vi "Boolean State Change.vi"(11 "Bool In":bool) -> (3 "State Change?":bool)   [LabVIEW 2018, in "Boolean Functions.lvlib"]
doc: "Detect change in state of the boolean input"
uses:
  Boolean Functions.lvlib
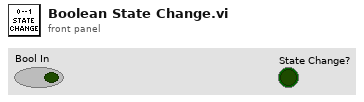
[diagram p1: front panel]
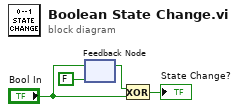
[diagram p0: block diagram]
diagram:
  n1 = feedback #1(FALSE ("Controller On?")) -> (w3:bool)
  n2 = feedback-in #1("Bool In") -> ()
  n3 = Exclusive Or(1:"Bool In", 2:w3) -> (0:→"State Change?":bool)
